vi "Calibration.vi"(8 "error in (no error)":errorcluster, 11 "Finish/Begin (Finish)":bool) -> (0 "error out":errorcluster)   [LabVIEW 2018]
doc: "This subVI enqueues the named action in to the communications queue along with the input data."
uses:
  Private Controls/Module Action.ctl
  Controller (Host).lvlib
  Private Controls/Module Data.ctl
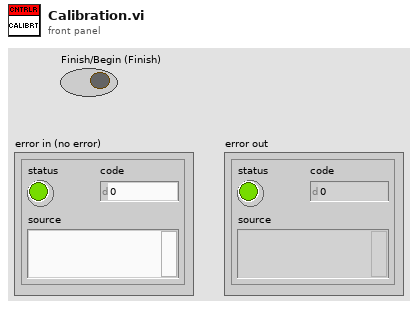
[diagram p1: front panel]
types:
  T1 = typedef "Controller (Host).lvlib/Module Data.ctl" = cluster{"Data":variant, "Action":T2}
  T2 = typedef "Controller (Host).lvlib/Module Action.ctl" = enum8{"Timeout", "Value to Monitor", "Init", "Reset Dev_Min_Max", "Error", "Exit", "Prompt Main Menu", "Prompt Test Info", "Prompt Operation Select", "Calibration", "Load APU Setup Data", "Update Report FilePath"}
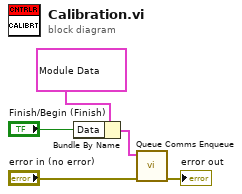
[diagram p0: block diagram]
diagram:
  n1 = Bundle By Name(cluster=T1 {"Data"=variant, "Action"=enum."Calibration"} ("element"), "Data"="Finish/Begin (Finish)") -> (w4:T1)
  n2 = call "Queue Comms Enqueue.vi"("error in (no error)"="error in (no error)", "element"=w4) -> ("error out"=→"error out":errorcluster)  [unwired: 9 in]
